vi "Senoide.vi"(1 "ruido":dbl, 2 "amplitude":dbl, 3 "variavel x":i32, 4 "taxa amostral":i32=3) -> (0 "saida":dbl[](array[numeric]))   [LabVIEW 2019]
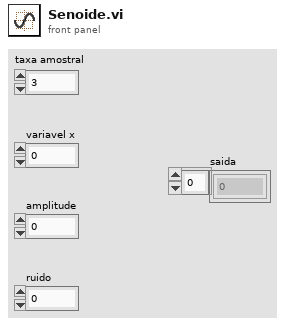
[diagram p1: front panel]
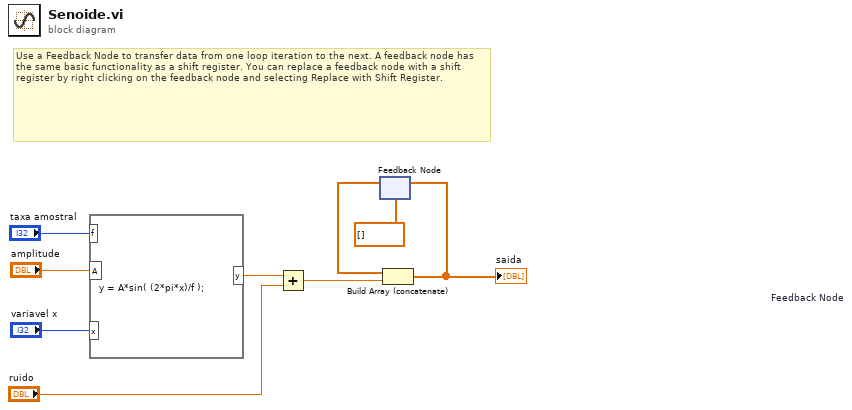
[diagram p0: block diagram]
diagram:
  # "Use a Feedback Node to transfer data from one loop iteration to the next. A feedback node has the same basic functionality as a shift register. You can replace a feedback node with a shift register by right clicking on the feedback node and selecting Replace with Shift Register."
  n1 = formula code="y = A*sin( (2*pi*x)/f );"("x"="variavel x", "f"="taxa amostral", "A"="amplitude") -> ("y"=w3:dbl)
  n2 = Add(x=w3, y="ruido") -> (x+y=w4:dbl)
  n3 = feedback #1 "Feedback Node"(dbl[] []) -> (w8:dbl[])
  n4 = Build Array (concatenate)(w8, w4) -> (w7:dbl[])
  "saida" <- w7
  n5 = feedback-in #1(w7) -> ()
